vi "Drive Controller.vi"(8 "error in":errorcluster) -> ()   [LabVIEW 2019]
doc: "This VI executes continuously carrying out the current operation and responding to updates or new operation requests. It will often contain the timing or control code that is difficult to place directly in TeleOp. This VI generally opens all sensors and motors and isolates the rest of the robot code from knowing implementation details of how the operations are carried out."
uses:
  <vilib>/Rock Robotics/WPI/Framework/Completion Status.ctl
  Drive Setpoints.ctl
  Drive Operations.ctl
  Drive Published Globals.vi
  <vilib>/addons/control/pid/pid.llb/PID (DBL).vi
  <vilib>/addons/control/pid/NI_PID_pid.lvlib
panel:
  out "Setpoints":T1(graph)
  in  "Motor CAN IDs":T2={"Left Leader"=1, "Left Follower 1"=2, "Left Follower 2"=3, "Right Leader"=5, "Right Follower 1"=6, "Right Follower 2"=7}
  in  "Interactive Values":T3
  in  "Buttons":cluster{"Execute Cmd":bool, "Abort Cmd":bool}
  out "Command Timing":cluster{"Start Time (ms)":u32, "Iterations":i32}
  out "Status":T5
  out "Current\nCmd":string
  # "Tip: The graph shows the motor setpoints. It may also be helpful to observe inputs and sensor values.\nYou may also want to display tuning or debugging controls."
  # "Click here to set min"
  # "Interactive Command: You may fill in the settings for a command\nand schedule it with the Execute button. You can observe and abort\nany command while fine tuning the code for the controller."
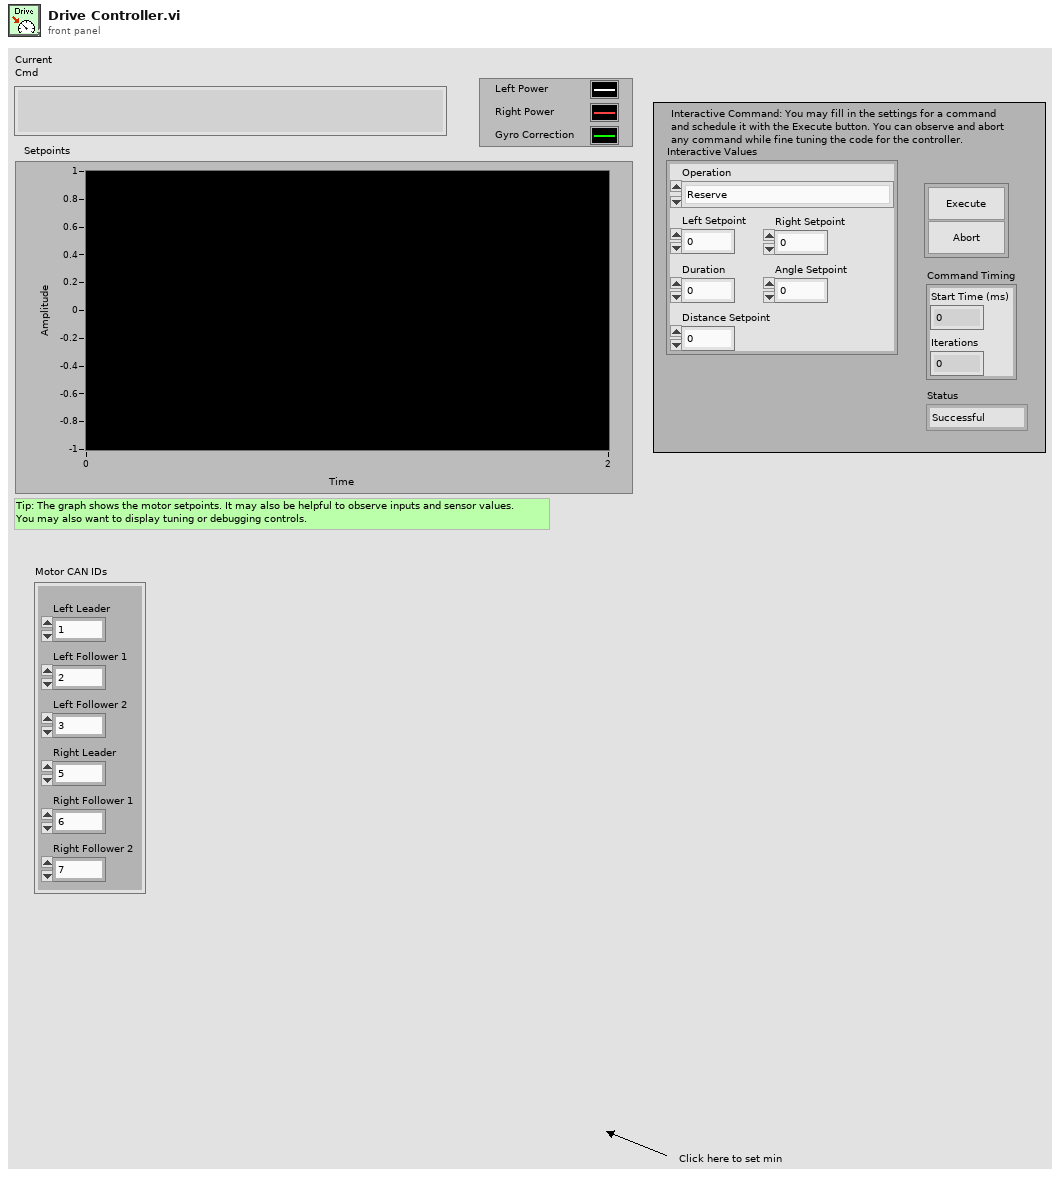
[diagram p1: front panel]
types:
  T1 = cluster{"output":dbl, "Left Setpoint":dbl, "output":dbl}
  T2 = cluster{"Left Leader":u8, "Left Follower 1":u8, "Left Follower 2":u8, "Right Leader":u8, "Right Follower 1":u8, "Right Follower 2":u8}
  T3 = typedef "Drive Setpoints.ctl" = cluster{"Operation":T4, "Left Setpoint":dbl, "Right Setpoint":dbl, "Duration":dbl, "Angle Setpoint":dbl, "Distance Setpoint":dbl}
  T4 = typedef "Drive Operations.ctl" = enum16{"Reserve", "Read Current", "Arcade Drive Immediate", "Arcade Drive Straight Immediate", "Drive for Time", "Turn to Angle", "Drive for Distance"}
  T5 = typedef "Completion Status.ctl" = enum16{"Successful", "Aborted", "Incomplete"}
  T6 = typedef "Command Status Info.ctl" = cluster{"Name":string, "Status":T5, "notifier out":T7}
  T7 = typedef "Completion Notifier.ctl" = refnum<notifier>
  T8 = cluster{"SubSystem Data":T3, cluster{"Start Time (ms)":u32, "Iterations":i32}, cluster{"Command Info":T6, "Description":string, "Default Command":T3, "queue out":refnum<queue>, "Subsystem Name":string}}
  T9 = typedef "WPI_MotorControlDeviceRef.ctl" = cluster{"DeviceStatus":errorcluster, "Type":T10, "PWM":cluster{"PWM Channel":T11, "DeadBand":T12}, "CAN":cluster{"Device Number":u8, "SetOutput VI Ref":variant, "GetOutput VI Ref":variant, "Enable VI Ref":variant, "Disable VI Ref":variant, "Data":variant}, "Invert":bool, "DIO PWM":cluster{"PWM \"Enable\" Channel":T11, "DIOChannel":T13, "PWM Rate":dbl}}
  T10 = typedef "WPI_MotorControlType.ctl" = enum16{"PWM", "CAN", "DIO PWM"}
  T11 = typedef "FPGA_DIOPWMChannel.ctl" = enum8{"PWM 0", "PWM 1", "PWM 2", "PWM 3", "PWM 4", "PWM 5", "PWM 6", "PWM 7", "PWM 8", "PWM 9", "PWM MXP 0", "PWM MXP 1", "PWM MXP 2", "PWM MXP 3", "PWM MXP 4", "PWM MXP 5", "PWM MXP 6", "PWM MXP 7", "PWM MXP 8", "PWM MXP 9", "Invalid"}
  T12 = typedef "WPI_PWMDeadband.ctl" = cluster{"Name":string, "maxPositivePwm":i32, "minPositivePwm":i32, "centerPwm":i32, "maxNegativePwm":i32, "minNegativePwm":i32, "angularRange":u16}
  T13 = typedef "FPGA_DIOChannel.ctl" = enum8{"DIO 0", "DIO 1", "DIO 2", "DIO 3", "DIO 4", "DIO 5", "DIO 6", "DIO 7", "DIO 8", "DIO 9", "DIO MXP 0", "DIO MXP 1", "DIO MXP 2", "DIO MXP 3", "DIO MXP 4", "DIO MXP 5", "DIO MXP 6", "DIO MXP 7", "DIO MXP 8", "DIO MXP 9", "DIO MXP 10", "DIO MXP 11", "DIO MXP 12", "DIO MXP 13", "DIO MXP 14", "DIO MXP 15", "SPI Port CS1", "SPI Port CS2", "SPI Port CS3", "SPI Port MISO", "SPI Port MOSI", "Invalid"}
  T14 = typedef "ADIS16448 Device Reference.ctl" = cluster{"DevStatus":errorcluster, "Hardware Config":T15, "Calibration Complete":refnum<notifier>, "Status FIFO":refnum<k33>, "Last Value Reference":refnum<data-value>, "Sychronous Process VI":T18, "Cmd FIFO":refnum<k33>, "Source":T19, "Data FIFO":refnum<k33>, "IMU Status LED Pin":T13, "Calibration Time":u32}
  T15 = typedef "ADIS16448 Hardware Configuration.ctl" = cluster{"SPI Clock Rate (Hz)":dbl, "IMU SPI Mode (3)":T16, "IMU Reset Pin":T13, "IMU SPI Bus":T17, "IMU Data Ready Pin":T13, "Stall Config":cluster{"Pow2BytesPerRead":u8, "StallTicks":u16, "CsToSclkTicks":u8}, "IMU Status LED Pin":T13}
  T16 = typedef "WPI_SPIMode.ctl" = enum16{"Mode 0 (Clk Idle Low,Sample on Leading)", "Mode 1 (Clk Idle Low,Sample on Trailing)", "Mode 2 (Clk Idle High,Sample on Leading)", "Mode 3 (Clk Idle High,Sample on Trailing)"}
  T17 = typedef "spi_bus.ctl" = enum16{"SPI On-Board, CS0", "SPI On-Board, CS1", "SPI On-Board, CS2", "SPI On-Board, CS3", "SPI MXP", "Invalid"}
  T18 = typedef "ADIS16448 Process.ctl" = refnum<vi>
  T19 = typedef "FPGA_CounterEncoderSourceConvertionLVSourceType.ctl" = cluster{"DevStatus":errorcluster, "AnalogTriggerMode?":bool, "DigitalMode":cluster{"DIO Channel":T20}, "AnalogTriggerMode":cluster{"AnalogTriggerIndex":T21, "OutputType":T22}}
  T20 = typedef "FPGA_DIODigitalSourceChannel.ctl" = enum8{"DIO 0", "DIO 1", "DIO 2", "DIO 3", "DIO 4", "DIO 5", "DIO 6", "DIO 7", "DIO 8", "DIO 9", "DIO MXP 0", "DIO MXP 1", "DIO MXP 2", "DIO MXP 3", "DIO MXP 4", "DIO MXP 5", "DIO MXP 6", "DIO MXP 7", "DIO MXP 8", "DIO MXP 9", "DIO MXP 10", "DIO MXP 11", "DIO MXP 12", "DIO MXP 13", "DIO MXP 14", "DIO MXP 15", "SPI Port CS1", "SPI Port CS2", "SPI Port CS3", "SPI Port MISO", "SPI Port MOSI", "Disabled"}
  T21 = typedef "FPGA_AnalogTriggerIndex.ctl" = enum8{"Trig 0", "Trig 1", "Trig 2", "Trig 3", "Trig 4", "Trig 5", "Trig 6", "Trig 7", "Invalid"}
  T22 = typedef "FPGA_AnalogTriggerOutType.ctl" = enum16{"InWindow", "TriggerState", "Rising", "Falling"}
  T23 = typedef "WPI_RobotDriveDevRef.ctl" = cluster{"DevStatus":errorcluster, "Motors[]":T9[], "Square Inputs":bool, "Max Output":dbl}
  T24 = typedef "ADIS16448 Data.ctl" = cluster{"XAngle":dbl, "YAngle":dbl, "ZAngle":dbl}
  T25 = cluster{"Left Power":dbl, "Right Power":dbl, "Gyro Correction":dbl}
  T26 = cluster{"proportional gain (Kc)":dbl, "integral time (Ti, min)":dbl, "derivative time (Td, min)":dbl}
  T27 = cluster{"SubSystem Data":T3, cluster{"Start Time (ms)":u32, "Iterations":i32}, "Default Command Arguments":cluster{"Command Info":T6, "Description":string, "Default Command":T3, "queue out":refnum<queue>, "Subsystem Name":string}}
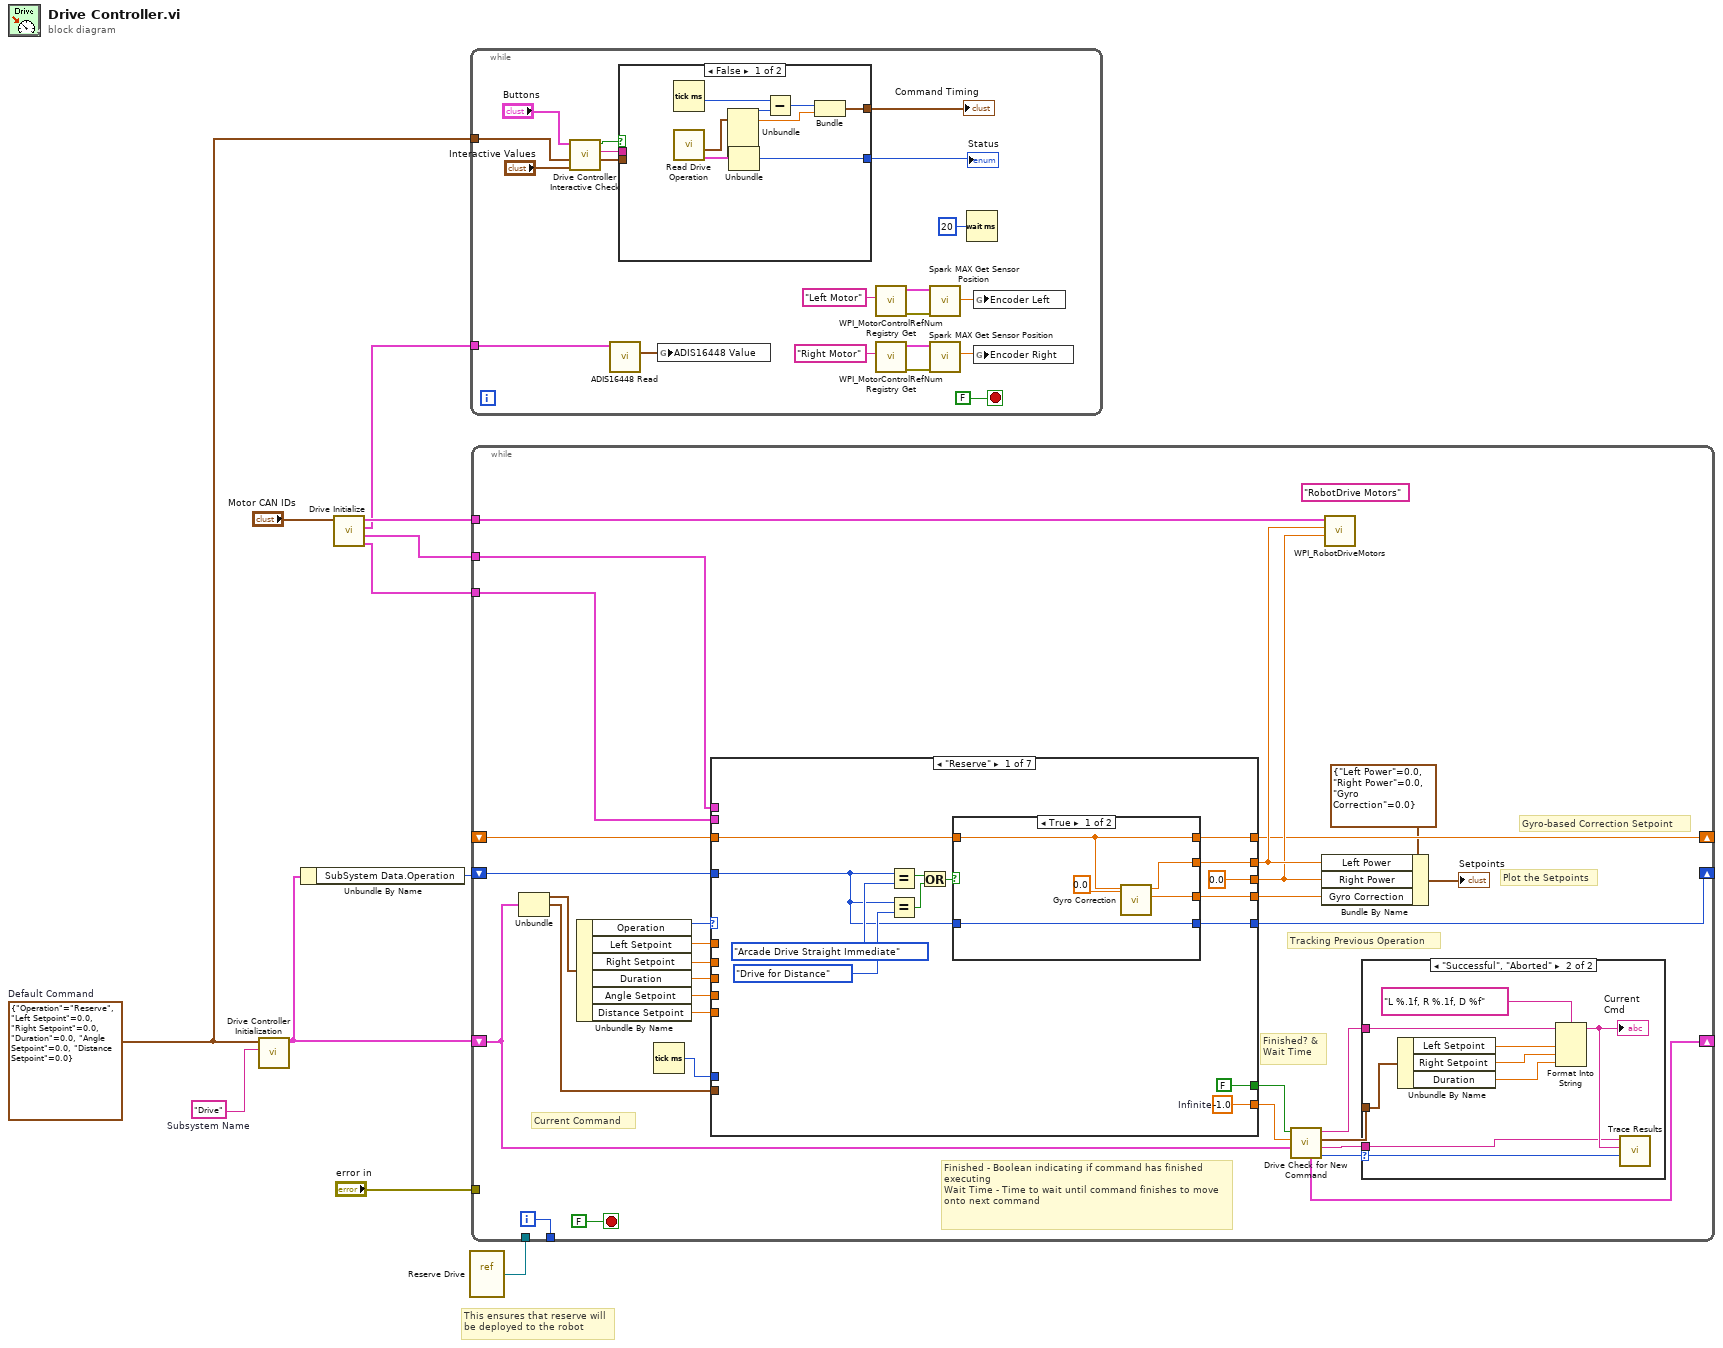
[diagram p0: block diagram]
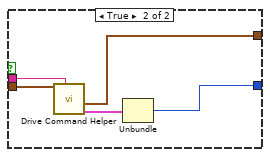
[diagram p2: hidden frame]
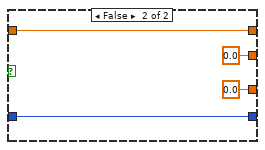
[diagram p4: hidden frame]
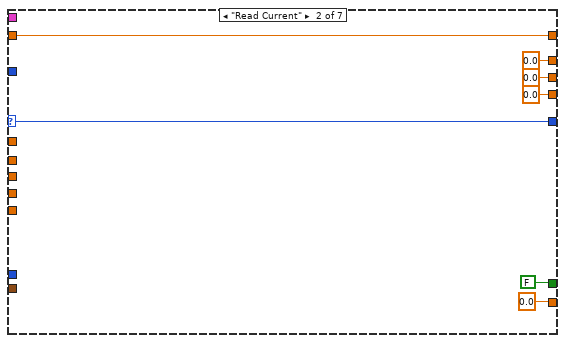
[diagram p5: hidden frame]
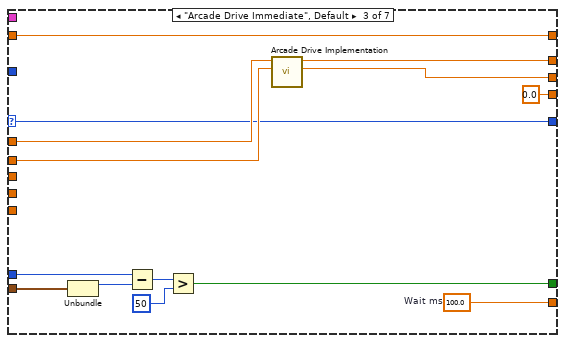
[diagram p6: hidden frame]
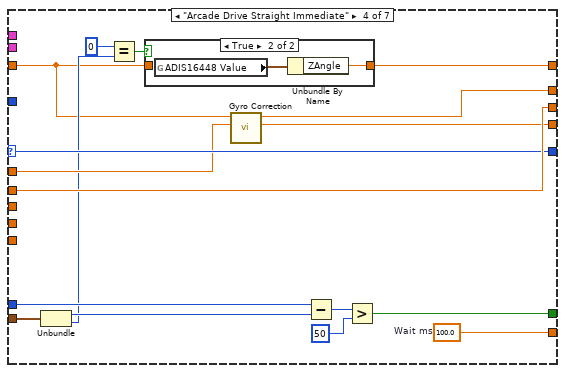
[diagram p7: hidden frame]
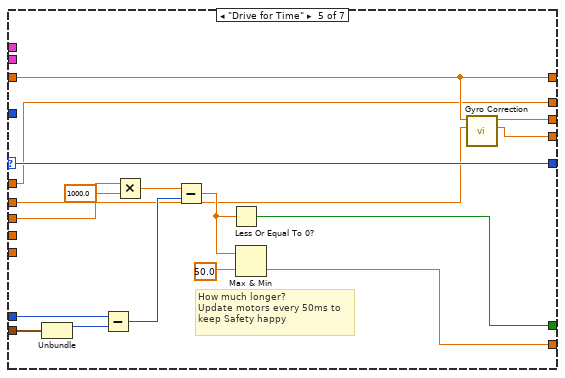
[diagram p9: hidden frame]
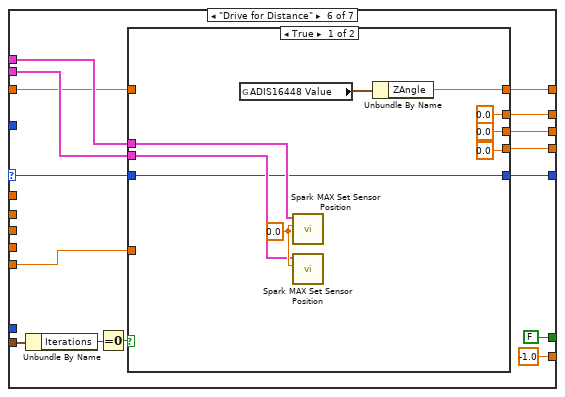
[diagram p10: hidden frame]
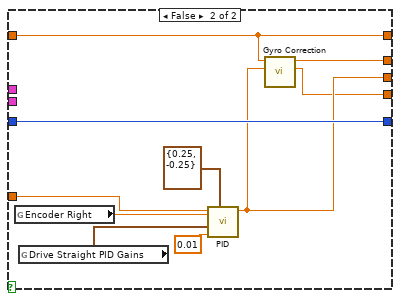
[diagram p11: hidden frame]
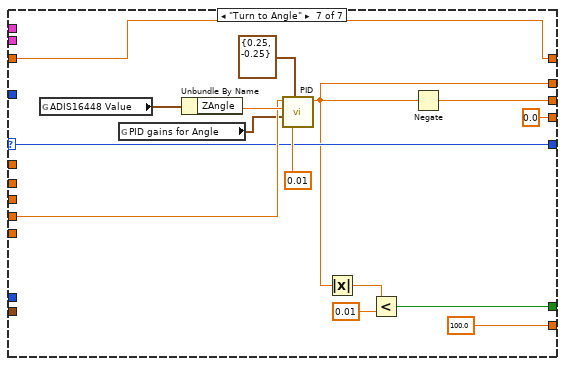
[diagram p12: hidden frame]
diagram:
  w3 = T3 {"Operation"=enum."Reserve", "Left Setpoint"=0.0, "Right Setpoint"=0.0, "Duration"=0.0, "Angle Setpoint"=0.0, "Distance Setpoint"=0.0}  # Default Command
  w11 = "Drive"  # Subsystem Name
  # "This ensures that reserve will\nbe deployed to the robot"
  n1 = call "Drive Controller Initialization.vi"("Subsystem Name"=w11, "Default Command"=w3) -> ("Current Command"=w5:T8)  [unwired: 9 in]
  n2 = Unbundle By Name(w5) -> ("SubSystem Data.Operation"=w4:T4)
  n3 = call "Drive Initialize.vi"("Motor CAN IDs"="Motor CAN IDs") -> ("Right Motor"=w1:T9, "Left Motor"=w2:T9, "imu"=w6:T14, "Drive"=w7:T23)  [unwired: 7 in]
  n4 = vi-ref "Reserve Drive.vi"() -> (w9:refnum<vi>)
  n5 = while {
    tunnel: w3 -> [w23]
    tunnel: w6 -> [w21]
    stop <- FALSE stop-if-true
    n6 = call "Drive Controller Interactive Check.vi"("Interactive Command In"="Interactive Values", "Default Command"=w23, "Buttons"="Buttons") -> ("Interactive Command Out"=w25:T3, "Trace String"=w26:string, "Schedule"=w27:bool)  [unwired: 6 in]
    n7 = call <vilib>:"ADIS16448 Read.vi"("ADIS16448DevRef"=w21) -> ("ADIS16448 Value"=w20:T24)  [unwired: 7 in, 3 out]
    n8 = case shown="False" w27 {
      tunnel: [w36 w44] -> w28
      tunnel: [w35 w40] -> w29
      tunnel: w26 -> [_ w42]
      tunnel: w25 -> [_ w41]
      frame False {
        n9 = Tick Count (ms)() -> (millisecond timer value=w39:u32)
        n10 = call "Read Drive Operation.vi"() -> ("Command Info"=w33:T6, "SubSystem Data"=w32:T3)  [unwired: 9 in, 1 out]
        n11 = Unbundle(w32) -> ("Operation"=w37:T4, "Left Setpoint"=w34:dbl)  [unwired: 4 out]
        n12 = Unbundle(w33) -> ("Status"=w36:T5)  [unwired: 2 out]
        n13 = Subtract(x=w39, y=w37) -> (x-y=w38:u32)
        n14 = Bundle(w38, "Left Setpoint"=w34) -> (w35:cluster{u32, "Left Setpoint":dbl})  [unwired: 1 in]
      }
      frame True {
        n15 = call "Drive Command Helper.vi"("Description"=w42, "SubSystem Data"=w41) -> ("Command Info Out"=w43:T6, "Command Timing"=w40:cluster{"Start Time (ms)":u32, "Iterations":i32})  [unwired: 7 in, 1 out]
        n16 = Unbundle(w43) -> ("Status"=w44:T5)  [unwired: 2 out]
      }
    }
    "Status" <- w28
    "Command Timing" <- w29
    n17 = global write "Drive Published Globals.vi" "ADIS16448 Value"(w20) -> ()
    n18 = call <vilib>:"WPI_MotorControlRefNum Registry Get.vi"("refnum name"="Left Motor") -> ("error out"=w19:errorcluster, "MotorControlDevRef"=w18:T9)  [unwired: 9 in]
    n19 = call <vilib>:"WPI_MotorControlRefNum Registry Get.vi"("refnum name"="Right Motor") -> ("error out"=w17:errorcluster, "MotorControlDevRef"=w16:T9)  [unwired: 9 in]
    n20 = call <vilib>:"Spark MAX Get Sensor Position.vi"("error in (no error)"=w19, "MotorControlDevRef in"=w18) -> ("Sensor Position"=w13:dbl)  [unwired: 6 in, 3 out]
    n21 = call <vilib>:"Spark MAX Get Sensor Position.vi"("error in (no error)"=w17, "MotorControlDevRef in"=w16) -> ("Sensor Position"=w12:dbl)  [unwired: 6 in, 3 out]
    n22 = Wait (ms)(milliseconds to wait=u32 20) -> ()  [unwired: 1 out]
    n23 = global write "Drive Published Globals.vi" "Encoder Left"(w13) -> ()
    n24 = global write "Drive Published Globals.vi" "Encoder Right"(w12) -> ()
  }
  n25 = while {
    shift-right: [w64] -> _
    shift-left: w5 -> [w57]
    tunnel: [w74] -> _
    tunnel: "error in" -> [_]
    tunnel: w9 -> [_]
    tunnel: w7 -> [w56]
    shift-right: [w54] -> _
    shift-left: w4 -> [w53]
    shift-right: [w52] -> _
    shift-left: _ -> [w51]
    tunnel: w2 -> [w50]
    tunnel: w1 -> [w48]
    i -> [w74]
    stop <- FALSE stop-if-true
    (unwired) "RobotDrive Motors" ("Name")
    # "Tracking Previous Operation"
    # "Gyro-based Correction Setpoint"
    # "Finished - Boolean indicating if command has finished executing\nWait Time - Time to wait until command finishes to move onto next command"
    # "Current Command"
    # "Plot the Setpoints"
    # "Finished? &\nWait Time"
    n26 = Unbundle(w57) -> ("SubSystem Data"=w71:T3, w58:cluster{"Start Time (ms)":u32, "Iterations":i32})  [unwired: 1 out]
    n27 = Unbundle By Name(w71) -> ("Operation"=w70:T4, "Left Setpoint"=w69:dbl, "Right Setpoint"=w68:dbl, "Duration"=w67:dbl, "Angle Setpoint"=w55:dbl, "Distance Setpoint"=w49:dbl)
    n28 = Tick Count (ms)() -> (millisecond timer value=w66:u32)
    n29 = case shown="\"Reserve\"" w70 {
      selector: w70 -> [_ w112 w117 w136 w154 w177 w207]
      tunnel: [w98 0.0 ("Wait ms") w122 w145 w155 -1.0 ("Wait ms") 100.0 ("Wait ms")] -> w63
      tunnel: [FALSE ("ignore previous (F)") FALSE ("ignore previous (F)") w123 w140 w160 FALSE ("ignore previous (F)") w203] -> w62
      tunnel: w58 -> [_ _ w126 w139 w162 w180 _]
      tunnel: [w85 0.0 ("output") w119 w137 w149 w168 w205] -> w73
      tunnel: [0.0 ("Left Setpoint") 0.0 ("output") w118 w138 w150 w167 w209] -> w72
      tunnel: w69 -> [_ _ w120 w135 w149 _ _]
      tunnel: w68 -> [_ _ w121 w138 w152 _ _]
      tunnel: w67 -> [_ _ _ _ w159 _ _]
      tunnel: w66 -> [_ _ w124 w141 w158 _ _]
      tunnel: w55 -> [_ _ _ _ _ _ w211]
      tunnel: [w96 w112 w117 w136 w154 w171 w207] -> w54
      tunnel: w53 -> [w89 _ _ _ _ _ _]
      tunnel: [w88 w111 w116 w134 w153 w173 w200] -> w52
      tunnel: w51 -> [w95 w111 w116 w130 w153 w174 w200]
      tunnel: w50 -> [_ _ _ _ _ w176 _]
      tunnel: w48 -> [_ _ _ _ _ w175 _]
      tunnel: w49 -> [_ _ _ _ _ w172 _]
      tunnel: [w86 0.0 ("output") 0.0 ("output") w129 w151 w166 0.0 ("output")] -> w45
      frame "Reserve" {
        w98 = -1.0  # Infinite
        n30 = Equal?(x=w89, y=Drive_Operations."Arcade Drive Straight Immediate") -> (x = y?=w93:bool)
        n31 = Equal?(x=w89, y=Drive_Operations."Drive for Distance") -> (x = y?=w91:bool)
        n32 = Or(x=w93, y=w91) -> (x .or. y?=w92:bool)
        n33 = case shown="True" w92 {
          tunnel: [w100 w106] -> w88
          tunnel: [w102 w107] -> w96
          tunnel: w95 -> [w100 w106]
          tunnel: w89 -> [w102 w107]
          tunnel: [w101 0.0 ("Correction")] -> w86
          tunnel: [w99 0.0 ("Corrected Setpoint")] -> w85
          frame True {
            n34 = call "Gyro Correction.vi"("Setpoint"=0.0 ("Left Setpoint"), "Angle Setpoint"=w100) -> ("Correction"=w101:dbl, "Corrected Setpoint"=w99:dbl)  [unwired: 8 in]
          }
          frame False {
          }
        }
      }
      frame "Read Current" {
      }
      frame "Arcade Drive Immediate", Default {
        w122 = 100.0  # Wait ms
        n35 = Unbundle(w126) -> ("Start Time (ms)"=w125:u32)  [unwired: 1 out]
        n36 = Subtract(x=w124, y=w125) -> (x-y=w127:u32)
        n37 = Greater?(x=w127, y=u8 50 ("Left Motor")) -> (0:w123:bool)
        n38 = call "Arcade Drive Implementation.vi"("Right Setpoint"=w121, "Left Setpoint"=w120) -> ("Numeric"=w118:dbl, "Numeric 2"=w119:dbl)  [unwired: 8 in]
      }
      frame "Arcade Drive Straight Immediate" {
        w145 = 100.0  # Wait ms
        n39 = Unbundle(w139) -> ("Start Time (ms)"=w142:u32, "Iterations"=w132:i32)
        n40 = Equal?(x=0, y=w132) -> (x = y?=w133:bool)
        n41 = case shown="True" w133 {
          tunnel: [w146 w147] -> w134
          tunnel: w130 -> [w146 _]
          frame False {
          }
          frame True {
            n42 = global read "Drive Published Globals.vi" "ADIS16448 Value"() -> (w148:T24)
            n43 = Unbundle By Name(w148) -> ("ZAngle"=w147:dbl)
          }
        }
        n44 = call "Gyro Correction.vi"("Setpoint"=w135, "Angle Setpoint"=w130) -> ("Correction"=w129:dbl, "Corrected Setpoint"=w137:dbl)  [unwired: 8 in]
        n45 = Subtract(x=w141, y=w142) -> (x-y=w143:u32)
        n46 = Greater?(x=w143, y=u8 50 ("Left Motor")) -> (0:w140:bool)
      }
      frame "Drive for Time" {
        # "How much longer?\nUpdate motors every 50ms to\nkeep Safety happy"
        n47 = Unbundle(w162) -> ("Start Time (ms)"=w161:u32)  [unwired: 1 out]
        n48 = Subtract(x=w158, y=w161) -> (x-y=w165:u32)
        n49 = Multiply(x=w159, y=1000.0) -> (x*y=w164:dbl)
        n50 = Subtract(x=w164, y=w165) -> (x-y=w157:dbl)
        n51 = Less Or Equal To 0?(x=w157) -> (x <= 0?=w160:bool)
        n52 = Max & Min(x=w157, y=50.0) -> (min(x,y)=w155:dbl)  [unwired: 1 out]
        n53 = call "Gyro Correction.vi"("Setpoint"=w152, "Angle Setpoint"=w153) -> ("Correction"=w151:dbl, "Corrected Setpoint"=w150:dbl)  [unwired: 8 in]
      }
      frame "Drive for Distance" {
        n54 = Unbundle By Name(w180) -> ("Iterations"=w170:i32)
        n55 = Equal To 0?(x=w170) -> (x = 0?=w169:bool)
        n56 = case shown="True" w169 {
          tunnel: w177 -> [w184 w195]
          tunnel: w176 -> [w188 _]
          tunnel: w175 -> [w187 _]
          tunnel: w174 -> [_ w193]
          tunnel: [w186 w193] -> w173
          tunnel: w172 -> [_ w199]
          tunnel: [0.0 ("output") w192] -> w167
          tunnel: [w184 w195] -> w171
          tunnel: [0.0 w191] -> w168
          tunnel: [0.0 ("Correction") w190] -> w166
          frame True {
            w189 = 0.0 ("Position")
            n57 = global read "Drive Published Globals.vi" "ADIS16448 Value"() -> (w185:T24)
            n58 = call <vilib>:"Spark MAX Set Sensor Position.vi"("Position"=w189, "MotorControlDeviceRef"=w188) -> ()  [unwired: 8 in, 2 out]
            n59 = call <vilib>:"Spark MAX Set Sensor Position.vi"("Position"=w189, "MotorControlDeviceRef"=w187) -> ()  [unwired: 8 in, 2 out]
            n60 = Unbundle By Name(w185) -> ("ZAngle"=w186:dbl)
          }
          frame False {
            n61 = global read "Drive Published Globals.vi" "Encoder Right"() -> (w194:dbl)
            n62 = global read "Drive Published Globals.vi" "Drive Straight PID Gains"() -> (w198:T26)
            n63 = call-poly <vilib>:"PID.vi"("output range"=cluster{"output high":dbl, "output low":dbl} {"output high"=0.25, "output low"=-0.25}, "dt (s)"=0.01, "PID gains"=w198, "process variable"=w194, "setpoint"=w199) -> ("output"=w192:dbl)  [unwired: 5 in, 1 out]
            n64 = call "Gyro Correction.vi"("Setpoint"=w192, "Angle Setpoint"=w193) -> ("Correction"=w190:dbl, "Corrected Setpoint"=w191:dbl)  [unwired: 8 in]
          }
        }
      }
      frame "Turn to Angle" {
        n65 = global read "Drive Published Globals.vi" "ADIS16448 Value"() -> (w213:T24)
        n66 = global read "Drive Published Globals.vi" "PID gains for Angle"() -> (w202:T26)
        n67 = Unbundle By Name(w213) -> ("ZAngle"=w212:dbl)
        n68 = call-poly <vilib>:"PID.vi"("output range"=cluster{"output high":dbl, "output low":dbl} {"output high"=0.25, "output low"=-0.25}, "dt (s)"=0.01, "PID gains"=w202, "process variable"=w212, "setpoint"=w211) -> ("output"=w205:dbl)  [unwired: 5 in, 1 out]
        n69 = Absolute Value(x=w205) -> (abs(x)=w204:dbl)
        n70 = Less?(x=w204, y=0.01) -> (x < y?=w203:bool)
        n71 = Negate(x=w205) -> (-x=w209:dbl)
      }
    }
    n72 = call "Drive Check for New Command.vi"("input cluster"=w57, "Wait time (ms)"=w63, "Finished?"=w62) -> ("Completion"=w65:T5, "Subsystem Name"=w59:string, "Current Command"=w60:T3, "Initial Trace String"=w61:string, "Next Command"=w64:T27)  [unwired: 4 in]
    n73 = Bundle By Name(cluster=T25 {"Left Power"=0.0, "Right Power"=0.0, "Gyro Correction"=0.0} ("Setpoints"), "Left Power"=w73, "Right Power"=w72, "Gyro Correction"=w45) -> (→"Setpoints":T25)
    n74 = call <vilib>:"WPI_RobotDriveMotors.vi"("RightSpeed"=w72, "LeftSpeed"=w73, "RobotDriveDevRef"=w56) -> ()  [unwired: 1 in, 8 out]
    n75 = case shown="\"Successful\", \"Aborted\"" w65 {
      selector: w65 -> [_ w84]
      tunnel: w61 -> [_ w79]
      tunnel: w60 -> [_ w80]
      tunnel: w59 -> [_ w76]
      frame "Incomplete", Default {
        # "Continuing current command"
      }
      frame "Successful", "Aborted" {
        # "Report and setup for next command"
        n76 = Unbundle By Name(w80) -> ("Left Setpoint"=w82:dbl, "Right Setpoint"=w83:dbl, "Duration"=w77:dbl)
        n77 = Format Into String(format string="L %.1f, R %.1f, D %f", initial string=w79, w82, w83, w77) -> (resulting string=w78:string)  [unwired: 1 in, 1 out]
        "Current\nCmd" <- w78
        n78 = call <vilib>:"Trace Results.vi"("Status of previous command"=w84, "Description"=w78, "Subsystem"=w76) -> ()  [unwired: 9 in]
      }
    }
  }
